vi "Host_SHVariables.vi"() -> ()   [LabVIEW 2019]
panel:
  out "Yeah_I_stopped":string
  in  "STOP":bool
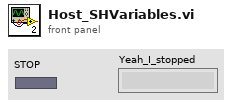
[diagram p1: front panel]
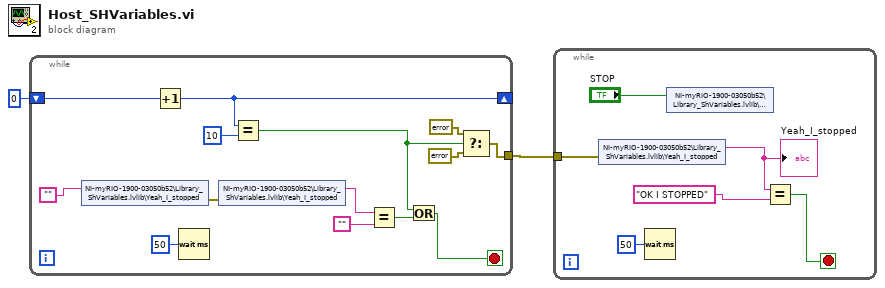
[diagram p0: block diagram]
diagram:
  n1 = while {
    tunnel: [w9] -> w1
    shift-right: [w14] -> _
    shift-left: u8 0 -> [w15]
    stop <- w12 stop-if-true
    n2 = shared-variable "NI-myRIO-1900-03050b52\\Library_ShVariables.lvlib\\Yeah_I_stopped"("") -> (error out=w3:errorcluster)  [unwired: 1 in]
    n3 = Increment(x=w15) -> (x+1=w14:u8)
    n4 = Wait (ms)(milliseconds to wait=u32 50) -> ()  [unwired: 1 out]
    n5 = shared-variable "NI-myRIO-1900-03050b52\\Library_ShVariables.lvlib\\Yeah_I_stopped"(error in=w3) -> (w5:string)  [unwired: 1 out]
    n6 = Equal?(x=w14, y=u8 10) -> (x = y?=w10:bool)
    n7 = Equal?(x=w5, y="") -> (x = y?=w11:bool)
    n8 = Or(x=w10, y=w11) -> (x .or. y?=w12:bool)
    n9 = Select(t=errorcluster {"status"=TRUE, "code"=0, "source"=""} ("error IO"), s=w10, f=errorcluster {"status"=FALSE, "code"=0, "source"=""} ("error IO")) -> (s? t:f=w9:errorcluster)
  }
  n10 = while {
    tunnel: w1 -> [w17]
    stop <- w21 stop-if-true
    n11 = shared-variable "NI-myRIO-1900-03050b52\\Library_ShVariables.lvlib\\Yeah_I_stopped"(error in=w17) -> (w18:string)  [unwired: 1 out]
    "Yeah_I_stopped" <- w18
    n12 = Wait (ms)(milliseconds to wait=u32 50) -> ()  [unwired: 1 out]
    n13 = shared-variable "NI-myRIO-1900-03050b52\\Library_ShVariables.lvlib\\StopSystem"("STOP") -> ()  [unwired: 1 in, 1 out]
    n14 = Equal?(x=w18, y="OK I STOPPED" ("Yeah_I_stopped")) -> (x = y?=w21:bool)
  }
